vi "Read Data.vi"(8 "error in (no error)":errorcluster, 11 "Exe Write in":refnum<class "Exe Write.lvclass">) -> (0 "error out":errorcluster, 2 "Base Data Lib:Data":refnum<class "Data.lvclass">, 3 "Exe Write out":refnum<class "Exe Write.lvclass">)   [LabVIEW 2016, in "File Library.lvlib" / "Exe Write.lvclass"]
uses:
  Exe Write.lvclass
  <vilib>/MSR Consulting, LLC/General Reuse/Data/Data.lvclass
  Exe Write.lvclass/Exe Write.ctl
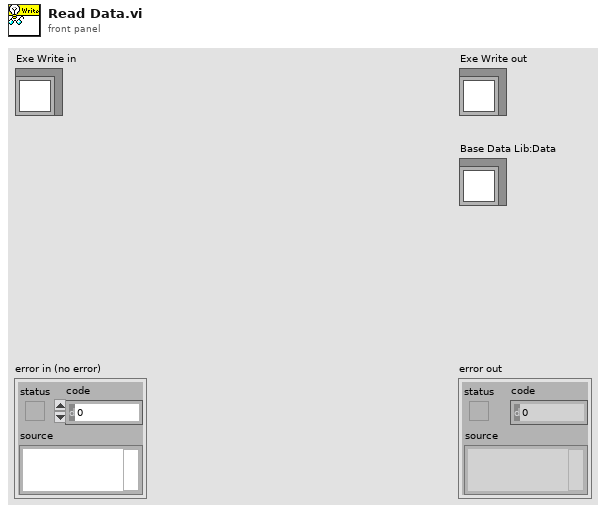
[diagram p1: front panel]
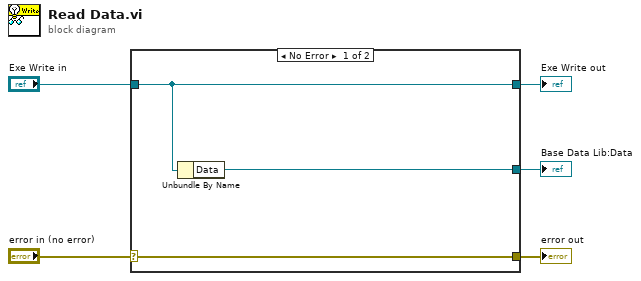
[diagram p0: block diagram]
diagram:
  n1 = case shown="No Error" "error in (no error)" {
    selector: "error in (no error)" -> [w8 w9]
    tunnel: [w8 w9] -> w4
    tunnel: [w7 w10] -> w2
    tunnel: "Exe Write in" -> [w7 w10]
    tunnel: [w6 _] -> w1
    frame No Error {
      n2 = Unbundle By Name(w7) -> ("Data"=w6:refnum<class "Data.lvclass">)
    }
    frame Error {
    }
  }
  "error out" <- w4
  "Exe Write out" <- w2
  "Base Data Lib:Data" <- w1
